vi "example_00_architecture.vi"() -> ()   [LabVIEW 2015, in "repub-dvr_nre.lvlib"]
uses:
  repub-dvr_nre.lvlib
  public/_controls/status.ctl
  public/_controls/configuration.ctl
  lv-recipe-machine/public/_controls/mode.ctl
  lv-recipe-machine/lv-recipe-machine.lvlib
  lv-recipe-machine/public/_controls/automatic_state.ctl
  lv-recipe-machine/public/_controls/manual_state.ctl
panel:
  in  "mode":T1
  in  "update_mode":bool
  out "error out":errorcluster
  in  "configuration":T2
  in  "Shutdown":bool
  in  "Initialize":bool
  in  "stop":bool
  out "status":T3
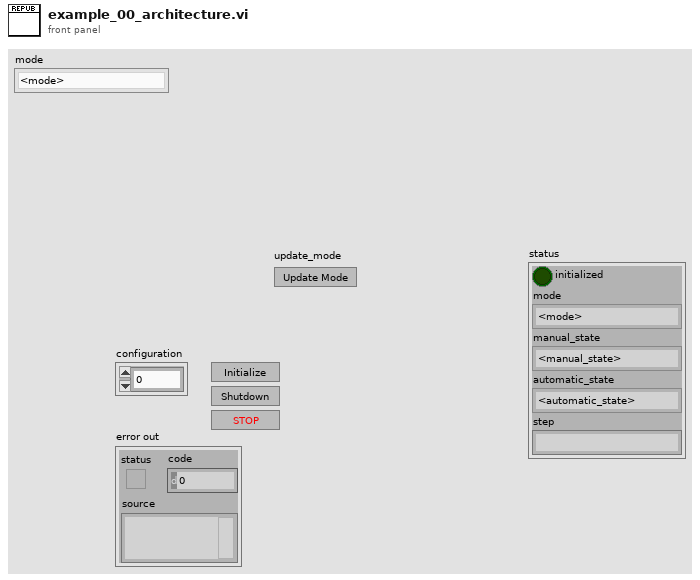
[diagram p1: front panel]
types:
  T1 = typedef "lv-recipe-machine.lvlib/mode.ctl" = enum16{"<mode>", "manual", "automatic", "<null>"}
  T2 = typedef "repub-dvr_nre.lvlib/configuration.ctl" = cluster{dbl}
  T3 = typedef "repub-dvr_nre.lvlib/status.ctl" = cluster{"initialized":bool, "mode":T1, "manual_state":T4, "automatic_state":T5, "step":string}
  T4 = typedef "lv-recipe-machine.lvlib/manual_state.ctl" = enum16{"<manual_state>", "failed", "action", "running", "idle", "<null>"}
  T5 = typedef "lv-recipe-machine.lvlib/automatic_state.ctl" = enum16{"<automatic_state>", "failed", "idle", "running", "paused", "transition", "stopped", "<null>"}
  T6 = typedef "repub-dvr_nre.lvlib/references.ctl" = cluster{"semaphore":T7, "input_queue":refnum<queue>, "output_queue":refnum<queue>, "data_dvr":refnum<data-value>, "stop_notifier":refnum<notifier>, "transition_queue":refnum<queue>, "change_in_notifier":refnum<notifier>, "change_out_notifier":refnum<notifier>, "change_in_event":refnum<user-event>, "change_out_event":refnum<user-event>}
  T7 = typedef "Semaphore RefNum" = refnum<k1>
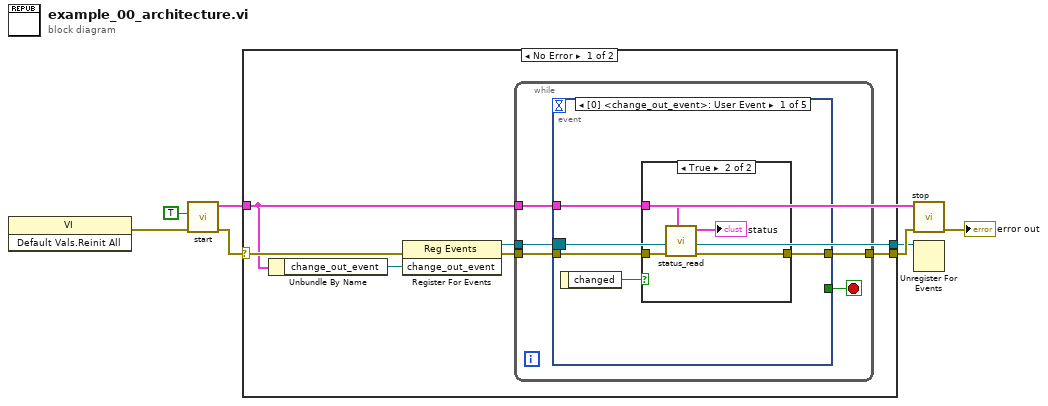
[diagram p0: block diagram]
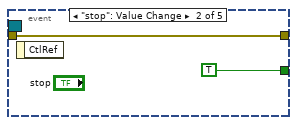
[diagram p3: hidden frame]
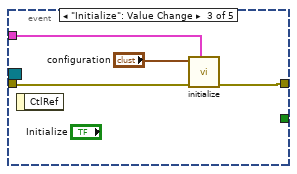
[diagram p4: hidden frame]
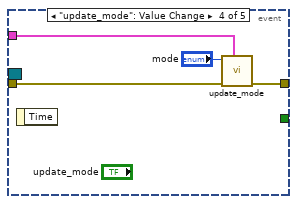
[diagram p5: hidden frame]
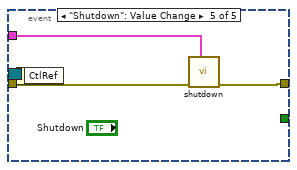
[diagram p6: hidden frame]
diagram:
  n1 = invoke class="VI" method="Default Vals.Reinit All"() -> (error out=w6:errorcluster)  [unwired: 3 in, 2 out]
  n2 = call "start.vi"("error in (no error)"=w6, "enable_event"=TRUE) -> ("error out"=w5:errorcluster, "references"=w4:T6)  [unwired: 8 in]
  n3 = case shown="No Error" w5 {
    selector: w5 -> [w12 w41]
    tunnel: [w13 w41] -> w7
    tunnel: w4 -> [w10 _]
    tunnel: [w8 _] -> w2
    frame No Error {
      n4 = Unbundle By Name(w10) -> ("change_out_event"=w9:refnum<user-event>)
      n5 = register-events(error in=w12, w9) -> (reference out=w8:refnum<event-registration>, error out=w11:errorcluster)  [unwired: 1 in]
      n6 = while {
        tunnel: w11 -> [w18]
        tunnel: [w17] -> w13
        tunnel: w10 -> [w15]
        tunnel: w8 -> [w14]
        stop <- w16 stop-if-true
        n7 = event shown="[0] <change_out_event>: User Event" {
          selector: w14 -> [_ _ _ _ _]
          dyn-events: _ -> [_ _ _ _ _]
          timeout: _ -> [_ _ _ _ _]
          tunnel: w18 -> [w22 w29 w30 w36 w38]
          tunnel: [w21 w29 w33 w37 w40] -> w17
          tunnel: [_ TRUE _ _ _] -> w16
          tunnel: w15 -> [w20 _ w31 w35 w39]
          event User Event {
            n8 = event-data() -> ("changed"=w19:bool)  [unwired: 1 in]
            n9 = case shown="True" w19 {
              tunnel: w22 -> [w23 w26]
              tunnel: [w23 w25] -> w21
              tunnel: w20 -> [_ w24]
              frame False {
              }
              frame True {
                n10 = call "status_read.vi"("references"=w24, "error in (no error)"=w26) -> ("error out"=w25:errorcluster, "status"=→"status":T3)  [unwired: 8 in]
              }
            }
          }
          event "stop": Value Change {
            n11 = event-data() -> ()  [unwired: 1 in, 1 out]
          }
          event "Initialize": Value Change {
            n12 = event-data() -> ()  [unwired: 1 in, 1 out]
            n13 = call "initialize.vi"("references"=w31, "error in (no error)"=w30, "configuration"="configuration") -> ("error out"=w33:errorcluster)  [unwired: 8 in]
          }
          event "update_mode": Value Change {
            n14 = event-data() -> ()  [unwired: 1 in, 1 out]
            n15 = call "update_mode.vi"("references"=w35, "error in (no error)"=w36, "mode"="mode") -> ("error out"=w37:errorcluster)  [unwired: 8 in]
          }
          event "Shutdown": Value Change {
            n16 = event-data() -> ()  [unwired: 1 in, 1 out]
            n17 = call "shutdown.vi"("references"=w39, "error in (no error)"=w38) -> ("error out"=w40:errorcluster)  [unwired: 9 in]
          }
        }
      }
    }
    frame Error {
    }
  }
  n18 = call "stop.vi"("error in (no error)"=w7, "references"=w4) -> ("error out"=→"error out":errorcluster)  [unwired: 9 in]
  n19 = Unregister For Events(event registration refnum=w2) -> ()  [unwired: 1 in, 1 out]
